vi "ExceptionStatus.vi"(8 "错误输入（无错误）":errorcluster, 9 "SocketQueue":T1, 10 "connection ID输入":refnum<k5>, 11 "socket 2":T2={"端口"=10013, "timeout"=10013, "标准差倍数"=0.0, "address"="{\"ad\":1}", "normal"="{\"ad\":0}"}) -> (0 "错误输出":errorcluster, 1 "connection ID输出":refnum<k5>)   [LabVIEW 2018]
uses:
  Initialize/Setting/SocketData.ctl
  Initialize/CreateQueue/SocketQueue.ctl
  <vilib>/Analysis/baseanly.llb/Mean (DBL).vi
  <vilib>/Analysis/NI_AALBase.lvlib
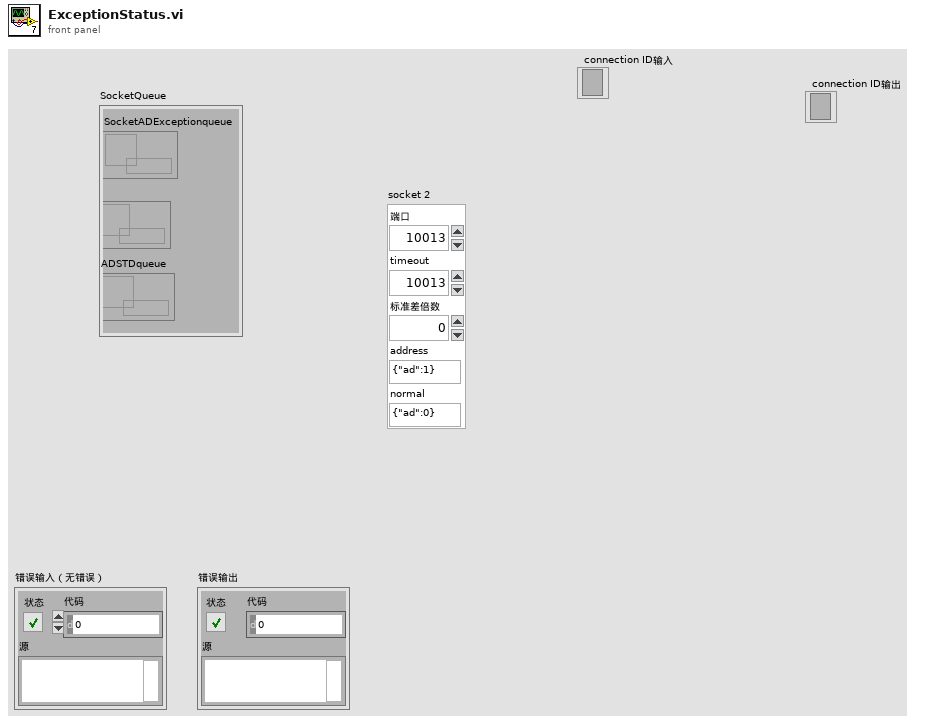
[diagram p1: front panel]
types:
  T1 = typedef "SocketQueue.ctl" = cluster{"ADSTDqueue ":refnum<queue>, "SocketADExceptionqueue":refnum<queue>, "  SocketAD":refnum<queue>}
  T2 = typedef "SocketData.ctl" = cluster{"端口":u16, "timeout":u16, "标准差倍数":dbl, "address":string, "normal":string}
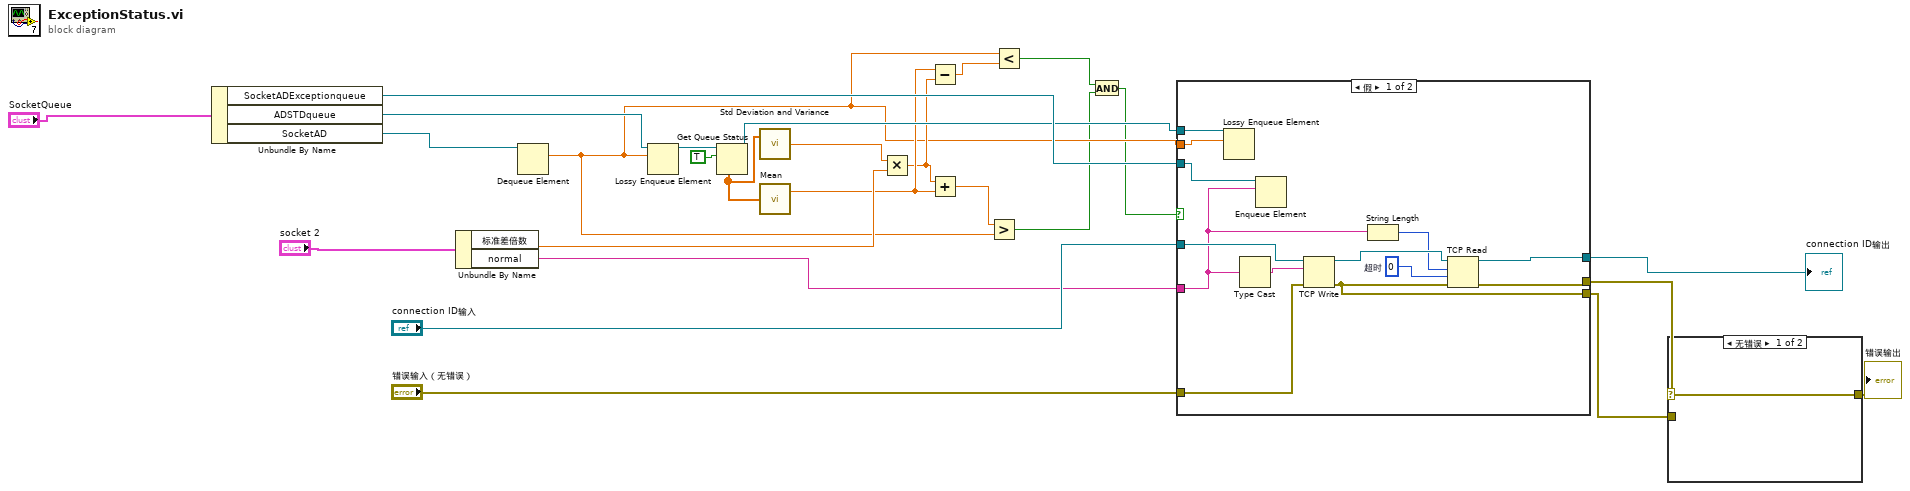
[diagram p0: block diagram]
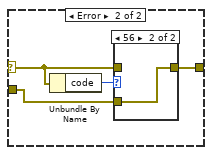
[diagram p2: hidden frame]
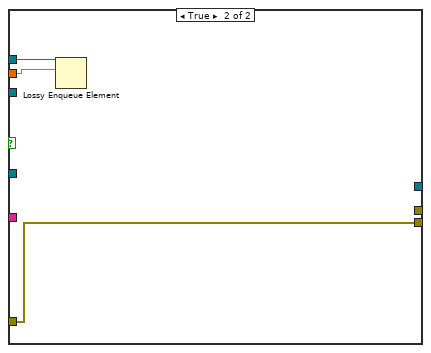
[diagram p4: hidden frame]
diagram:
  n1 = Unbundle By Name("SocketQueue") -> ("SocketADExceptionqueue"=w14:refnum<queue>, "ADSTDqueue"=w18:refnum<queue>, "SocketAD"=w13:refnum<queue>)
  n2 = Unbundle By Name("socket 2") -> ("标准差倍数"=w11:dbl, "normal"=w16:string)
  n3 = Dequeue Element(queue=w13) -> (element=w5:dbl)  [unwired: 2 in, 3 out]
  n4 = Lossy Enqueue Element(queue=w18, element=w5) -> (queue out=w19:refnum<queue>)  [unwired: 1 in, 3 out]
  n5 = Get Queue Status(queue=w19, return elements? (F)=TRUE ("返回元素？(F)")) -> (queue out=w8:refnum<queue>, elements=w17:dbl[])  [unwired: 1 in, 6 out]
  n6 = call <vilib>:"Std Deviation and Variance.vi"("X"=w17) -> ("standard deviation"=w12:dbl)  [unwired: 1 in, 2 out]
  n7 = call-poly <vilib>:"Mean.vi"("X"=w17) -> ("mean"=w7:dbl)  [unwired: 1 out]
  n8 = Multiply(x=w12, y=w11) -> (x*y=w6:dbl)
  n9 = Subtract(x=w7, y=w6) -> (x-y=w4:dbl)
  n10 = Add(x=w6, y=w7) -> (x+y=w10:dbl)
  n11 = Greater?(x=w10, y=w5) -> (0:w2:bool)
  n12 = Less?(x=w5, y=w4) -> (x < y?=w3:bool)
  n13 = And(x=w3, y=w2) -> (x .and. y?=w1:bool)
  n14 = case shown="假" w1 {
    tunnel: "connection ID输入" -> [w35 _]
    tunnel: [w34 _] -> w24
    tunnel: [w32 _] -> w26
    tunnel: [w33 w42] -> w23
    tunnel: "错误输入（无错误）" -> [w36 w42]
    tunnel: w14 -> [w31 _]
    tunnel: w16 -> [w30 _]
    tunnel: w8 -> [w28 w41]
    tunnel: w5 -> [w27 w40]
    frame False {
      w39 = 0  # 超时
      n15 = Lossy Enqueue Element(queue=w28, element=w27) -> ()  [unwired: 1 in, 4 out]
      n16 = Type Cast(x=w30) -> (*(type *) &x=w38:string)  [unwired: 1 out]
      n17 = Enqueue Element(queue=w31, element=w30) -> ()  [unwired: 2 in, 3 out]
      n18 = TCP Write(connection ID=w35, data in=w38, error in (no error)=w36) -> (connection ID out=w37:refnum<k5>, error out=w33:errorcluster)  [unwired: 2 out]
      n19 = String Length(string=w30) -> (length=w29:i32)
      n20 = TCP Read(connection ID=w37, bytes to read=w29, error in (no error)=w33, 9:w39) -> (connection ID out=w32:refnum<k5>, error out=w34:errorcluster)  [unwired: 1 in, 1 out]
    }
    frame True {
      n21 = Lossy Enqueue Element(queue=w41, element=w40) -> ()  [unwired: 1 in, 4 out]
    }
  }
  "connection ID输出" <- w26
  n22 = case shown="无错误" w24 {
    selector: w24 -> [w43 w46]
    tunnel: [w43 w44] -> w25
    tunnel: w23 -> [_ w45]
    frame No Error {
    }
    frame Error {
      n23 = Unbundle By Name(w46) -> ("code"=w47:i32)
      n24 = case shown="56" w47 {
        tunnel: w46 -> [w48 _]
        tunnel: w45 -> [_ w49]
        tunnel: [w48 w49] -> w44
        frame Default {
        }
        frame 56 {
        }
      }
    }
  }
  "错误输出" <- w25
